vi "Finish.vi"   [LabVIEW 2016]
doc: "This VI is called just before exiting. It is expected to close I/O refnum, save collected data, etc."
uses:
  <vilib>/Rock Robotics/WPI/Utilities/WPI_GetSetVariantRefNum.vi
types:
  T1 = typedef "WPI_JoystickDevRef.ctl" = cluster{"Device":T2}
  T2 = typedef "WPI_JoystickDeviceEnum.ctl" = enum16{"USB 0", "USB 1", "USB 2", "USB 3", "USB 4", "USB 5"}
  T3 = typedef "WPI_MotorControlDeviceRef.ctl" = cluster{"DeviceStatus":errorcluster, "Type":T4, "PWM":cluster{"PWM Channel":T5, "DeadBand":T6}, "CAN":cluster{"Device Number":u8, "SetOutput VI Ref":variant, "GetOutput VI Ref":variant, "Enable VI Ref":variant, "Disable VI Ref":variant, "Data":variant}, "Invert":bool}
  T4 = typedef "WPI_MotorControlType.ctl" = enum16{"PWM", "CAN"}
  T5 = typedef "FPGA_DIOPWMChannel.ctl" = enum8{"PWM 0", "PWM 1", "PWM 2", "PWM 3", "PWM 4", "PWM 5", "PWM 6", "PWM 7", "PWM 8", "PWM 9", "PWM MXP 0", "PWM MXP 1", "PWM MXP 2", "PWM MXP 3", "PWM MXP 4", "PWM MXP 5", "PWM MXP 6", "PWM MXP 7", "PWM MXP 8", "PWM MXP 9", "Invalid"}
  T6 = typedef "WPI_PWMDeadband.ctl" = cluster{"Name":string, "maxPositivePwm":i32, "minPositivePwm":i32, "centerPwm":i32, "maxNegativePwm":i32, "minNegativePwm":i32, "angularRange":u16}
  T7 = typedef "WPI_CounterDevRef.ctl" = cluster{"DevStatus":errorcluster, "CntIndex":T8}
  T8 = typedef "FPGA_CounterCtrSystemIndex.ctl" = enum8{"Ctr 0", "Ctr 1", "Ctr 2", "Ctr 3", "Ctr 4", "Ctr 5", "Ctr 6", "Ctr 7", "Invalid"}
  T9 = typedef "WPI_EncoderDevRef.ctl" = cluster{"DevStatus":errorcluster, "EncoderIndex":T10, "CounterIndex":T8, "DistancePerCount":dbl, "Decoding Type":T11}
  T10 = typedef "FPGA_EncoderIdx.ctl" = enum8{"Enc 0", "Enc 1", "Enc 2", "Enc 3", "Enc 4", "Enc 5", "Enc 6", "Enc 7", "Invalid"}
  T11 = typedef "WPI_EncoderType.ctl" = enum16{"1x", "2x", "4x"}
  T12 = typedef "WPI_DigitalInputDevRef.ctl" = cluster{"DevStatus":errorcluster, "DIO Channel":T13}
  T13 = typedef "FPGA_DIOChannel.ctl" = enum8{"DIO 0", "DIO 1", "DIO 2", "DIO 3", "DIO 4", "DIO 5", "DIO 6", "DIO 7", "DIO 8", "DIO 9", "DIO MXP 0", "DIO MXP 1", "DIO MXP 2", "DIO MXP 3", "DIO MXP 4", "DIO MXP 5", "DIO MXP 6", "DIO MXP 7", "DIO MXP 8", "DIO MXP 9", "DIO MXP 10", "DIO MXP 11", "DIO MXP 12", "DIO MXP 13", "DIO MXP 14", "DIO MXP 15", "SPI Port CS1", "SPI Port CS2", "SPI Port CS3", "SPI Port MISO", "SPI Port MOSI", "Invalid"}
  T14 = typedef "WPI_RobotDriveDevRef.ctl" = cluster{"DevStatus":errorcluster, "Motors[]":T3[], "Square Inputs":bool, "Max Output":dbl}
  T15 = typedef "WPI_SolenoidDevRef.ctl" = cluster{"DevStatus":errorcluster, "Pneumatics Control Module":u8, "Forward Solenoid Channel":T16, "Reverse Solenoid Channel":T16}
  T16 = typedef "WPI_SolenoidChannel.ctl" = enum8{"Solenoid 0", "Solenoid 1", "Solenoid 2", "Solenoid 3", "Solenoid 4", "Solenoid 5", "Solenoid 6", "Solenoid 7", "Invalid"}
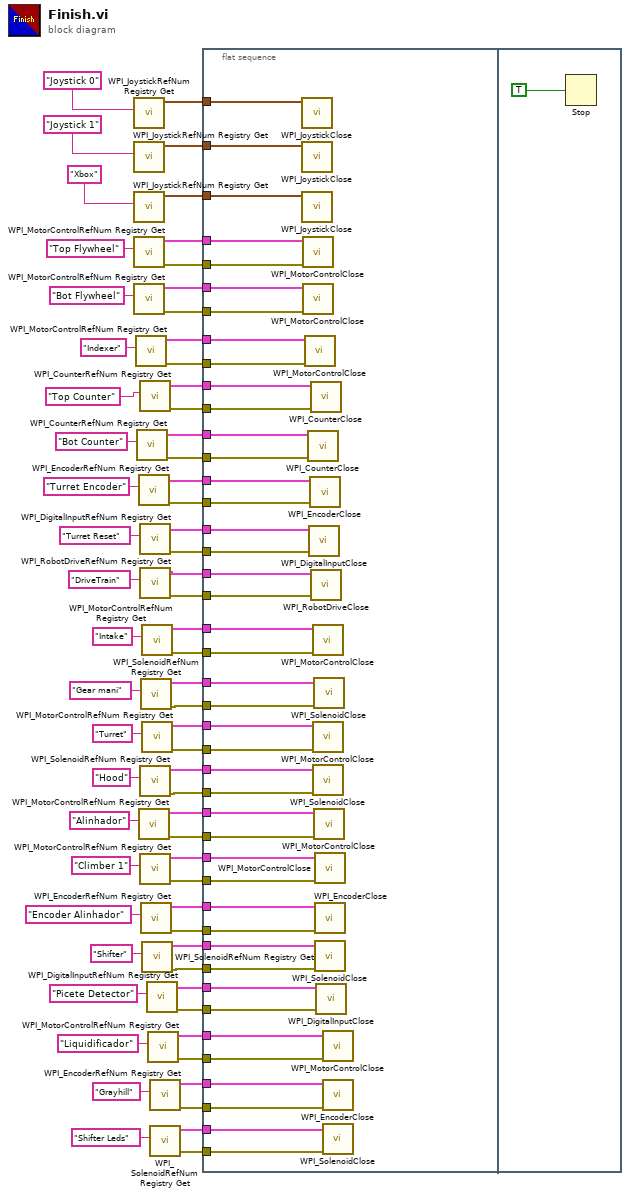
[diagram p0: block diagram]
diagram:
  n1 = call <vilib>:"WPI_JoystickRefNum Registry Get.vi"("refnum name"="Joystick 0") -> ("JoystickDevRef"=w65:T1)  [unwired: 1 in, 9 out]
  n2 = call <vilib>:"WPI_JoystickRefNum Registry Get.vi"("refnum name"="Joystick 1") -> ("JoystickDevRef"=w64:T1)  [unwired: 1 in, 9 out]
  n3 = call <vilib>:"WPI_JoystickRefNum Registry Get.vi"("refnum name"="Xbox") -> ("JoystickDevRef"=w61:T1)  [unwired: 1 in, 9 out]
  n4 = call <vilib>:"WPI_MotorControlRefNum Registry Get.vi"("refnum name"="Top Flywheel") -> ("error out"=w59:errorcluster, "MotorControlDevRef"=w60:T3)  [unwired: 9 in]
  n5 = call <vilib>:"WPI_MotorControlRefNum Registry Get.vi"("refnum name"="Bot Flywheel") -> ("error out"=w56:errorcluster, "MotorControlDevRef"=w55:T3)  [unwired: 9 in]
  n6 = call <vilib>:"WPI_MotorControlRefNum Registry Get.vi"("refnum name"="Indexer") -> ("error out"=w53:errorcluster, "MotorControlDevRef"=w54:T3)  [unwired: 9 in]
  n7 = call <vilib>:"WPI_CounterRefNum Registry Get.vi"("refnum name"="Bot Counter") -> ("error out"=w50:errorcluster, "CounterDevRef"=w49:T7)  [unwired: 9 in]
  n8 = call <vilib>:"WPI_EncoderRefNum Registry Get.vi"("refnum name"="Turret Encoder") -> ("error out"=w47:errorcluster, "EncoderDevRef"=w48:T9)  [unwired: 9 in]
  n9 = call <vilib>:"WPI_MotorControlRefNum Registry Get.vi"("refnum name"="Alinhador") -> ("error out"=w24:errorcluster, "MotorControlDevRef"=w25:T3)  [unwired: 9 in]
  n10 = call <vilib>:"WPI_CounterRefNum Registry Get.vi"("refnum name"="Top Counter") -> ("error out"=w2:errorcluster, "CounterDevRef"=w3:T7)  [unwired: 9 in]
  n11 = call <vilib>:"WPI_DigitalInputRefNum Registry Get.vi"("refnum name"="Turret Reset") -> ("error out"=w43:errorcluster, "DigitalInputDevRef"=w44:T12)  [unwired: 9 in]
  n12 = call <vilib>:"WPI_RobotDriveRefNum Registry Get.vi"("refnum name"="DriveTrain") -> ("error out"=w41:errorcluster, "RobotDriveDevRef"=w42:T14)  [unwired: 9 in]
  n13 = call <vilib>:"WPI_SolenoidRefNum Registry Get.vi"("refnum name"="Hood") -> ("error out"=w29:errorcluster, "SolenoidDevRef"=w28:T15)  [unwired: 9 in]
  n14 = call <vilib>:"WPI_MotorControlRefNum Registry Get.vi"("refnum name"="Climber 1") -> ("error out"=w22:errorcluster, "MotorControlDevRef"=w23:T3)  [unwired: 9 in]
  n15 = call <vilib>:"WPI_SolenoidRefNum Registry Get.vi"("refnum name"="Gear mani") -> ("error out"=w35:errorcluster, "SolenoidDevRef"=w36:T15)  [unwired: 9 in]
  n16 = call <vilib>:"WPI_EncoderRefNum Registry Get.vi"("refnum name"="Encoder Alinhador") -> ("error out"=w19:errorcluster, "EncoderDevRef"=w20:T9)  [unwired: 9 in]
  n17 = call <vilib>:"WPI_MotorControlRefNum Registry Get.vi"("refnum name"="Intake") -> ("error out"=w38:errorcluster, "MotorControlDevRef"=w39:T3)  [unwired: 9 in]
  n18 = call <vilib>:"WPI_MotorControlRefNum Registry Get.vi"("refnum name"="Turret") -> ("error out"=w32:errorcluster, "MotorControlDevRef"=w31:T3)  [unwired: 9 in]
  n19 = call <vilib>:"WPI_SolenoidRefNum Registry Get.vi"("refnum name"="Shifter") -> ("error out"=w17:errorcluster, "SolenoidDevRef"=w18:T15)  [unwired: 9 in]
  n20 = call <vilib>:"WPI_DigitalInputRefNum Registry Get.vi"("refnum name"="Picete Detector") -> ("error out"=w15:errorcluster, "DigitalInputDevRef"=w14:T12)  [unwired: 9 in]
  n21 = call <vilib>:"WPI_MotorControlRefNum Registry Get.vi"("refnum name"="Liquidificador") -> ("error out"=w12:errorcluster, "MotorControlDevRef"=w11:T3)  [unwired: 9 in]
  n22 = call <vilib>:"WPI_EncoderRefNum Registry Get.vi"("refnum name"="Grayhill") -> ("error out"=w8:errorcluster, "EncoderDevRef"=w9:T9)  [unwired: 9 in]
  n23 = call <vilib>:"WPI_SolenoidRefNum Registry Get.vi"("refnum name"="Shifter Leds") -> ("error out"=w5:errorcluster, "SolenoidDevRef"=w6:T15)  [unwired: 9 in]
  n24 = flat-sequence {
    tunnel: w65 -> [w109]
    tunnel: w64 -> [w108]
    tunnel: w61 -> [w107]
    tunnel: w60 -> [w105]
    tunnel: w59 -> [w106]
    tunnel: w55 -> [w104]
    tunnel: w56 -> [w103]
    tunnel: w54 -> [w101]
    tunnel: w53 -> [w102]
    tunnel: w49 -> [w99]
    tunnel: w50 -> [w100]
    tunnel: w48 -> [w98]
    tunnel: w47 -> [w97]
    tunnel: w44 -> [w96]
    tunnel: w43 -> [w95]
    tunnel: w42 -> [w94]
    tunnel: w41 -> [w93]
    tunnel: w39 -> [w92]
    tunnel: w38 -> [w91]
    tunnel: w36 -> [w90]
    tunnel: w35 -> [w89]
    tunnel: w31 -> [w87]
    tunnel: w32 -> [w88]
    tunnel: w28 -> [w85]
    tunnel: w29 -> [w86]
    tunnel: w25 -> [w84]
    tunnel: w24 -> [w83]
    tunnel: w23 -> [w82]
    tunnel: w22 -> [w81]
    tunnel: w20 -> [w80]
    tunnel: w19 -> [w79]
    tunnel: w18 -> [w78]
    tunnel: w17 -> [w77]
    tunnel: w14 -> [w75]
    tunnel: w15 -> [w76]
    tunnel: w11 -> [w73]
    tunnel: w12 -> [w74]
    tunnel: w9 -> [w72]
    tunnel: w8 -> [w71]
    tunnel: w6 -> [w70]
    tunnel: w5 -> [w69]
    tunnel: w3 -> [w68]
    tunnel: w2 -> [w67]
    frame #0 {
      n25 = call <vilib>:"WPI_JoystickClose.vi"("JoystickDevRef"=w109) -> ()  [unwired: 11 out]
      n26 = call <vilib>:"WPI_JoystickClose.vi"("JoystickDevRef"=w108) -> ()  [unwired: 11 out]
      n27 = call <vilib>:"WPI_JoystickClose.vi"("JoystickDevRef"=w107) -> ()  [unwired: 11 out]
      n28 = call <vilib>:"WPI_MotorControlClose.vi"("error in"=w106, "MotorControlDevRef"=w105) -> ()  [unwired: 9 in, 1 out]
      n29 = call <vilib>:"WPI_MotorControlClose.vi"("error in"=w103, "MotorControlDevRef"=w104) -> ()  [unwired: 9 in, 1 out]
      n30 = call <vilib>:"WPI_MotorControlClose.vi"("error in"=w102, "MotorControlDevRef"=w101) -> ()  [unwired: 9 in, 1 out]
      n31 = call <vilib>:"WPI_CounterClose.vi"("error in (no error)"=w100, "CounterDevRef"=w99) -> ()  [unwired: 9 in, 1 out]
      n32 = call <vilib>:"WPI_DigitalInputClose.vi"("error in (no error)"=w95, "DigitalInputDevRef"=w96) -> ()  [unwired: 9 in, 1 out]
      n33 = call <vilib>:"WPI_EncoderClose.vi"("error in (no error)"=w97, "EncoderDevRef"=w98) -> ()  [unwired: 9 in, 1 out]
      n34 = call <vilib>:"WPI_CounterClose.vi"("error in (no error)"=w67, "CounterDevRef"=w68) -> ()  [unwired: 9 in, 1 out]
      n35 = call <vilib>:"WPI_RobotDriveClose.vi"("error in (no error)"=w93, "RobotDriveDevRef"=w94) -> ()  [unwired: 9 in, 1 out]
      n36 = call <vilib>:"WPI_MotorControlClose.vi"("error in"=w91, "MotorControlDevRef"=w92) -> ()  [unwired: 9 in, 1 out]
      n37 = call <vilib>:"WPI_MotorControlClose.vi"("error in"=w88, "MotorControlDevRef"=w87) -> ()  [unwired: 9 in, 1 out]
      n38 = call <vilib>:"WPI_SolenoidClose.vi"("error in (no error)"=w86, "SolenoidDevRef"=w85) -> ()  [unwired: 9 in, 1 out]
      n39 = call <vilib>:"WPI_SolenoidClose.vi"("error in (no error)"=w89, "SolenoidDevRef"=w90) -> ()  [unwired: 9 in, 1 out]
      n40 = call <vilib>:"WPI_MotorControlClose.vi"("error in"=w83, "MotorControlDevRef"=w84) -> ()  [unwired: 9 in, 1 out]
      n41 = call <vilib>:"WPI_MotorControlClose.vi"("error in"=w81, "MotorControlDevRef"=w82) -> ()  [unwired: 9 in, 1 out]
      n42 = call <vilib>:"WPI_EncoderClose.vi"("error in (no error)"=w79, "EncoderDevRef"=w80) -> ()  [unwired: 9 in, 1 out]
      n43 = call <vilib>:"WPI_SolenoidClose.vi"("error in (no error)"=w77, "SolenoidDevRef"=w78) -> ()  [unwired: 9 in, 1 out]
      n44 = call <vilib>:"WPI_DigitalInputClose.vi"("error in (no error)"=w76, "DigitalInputDevRef"=w75) -> ()  [unwired: 9 in, 1 out]
      n45 = call <vilib>:"WPI_MotorControlClose.vi"("error in"=w74, "MotorControlDevRef"=w73) -> ()  [unwired: 9 in, 1 out]
      n46 = call <vilib>:"WPI_EncoderClose.vi"("error in (no error)"=w71, "EncoderDevRef"=w72) -> ()  [unwired: 9 in, 1 out]
      n47 = call <vilib>:"WPI_SolenoidClose.vi"("error in (no error)"=w69, "SolenoidDevRef"=w70) -> ()  [unwired: 9 in, 1 out]
    }
    frame #1 {
      n48 = Stop(stop? (T)=TRUE ("Quit")) -> ()
    }
  }
